vi "Stepper Configure.vi"(7 "Stepper #":u8, 8 "Error In":errorcluster, 9 "Control Method":T4=enum."2 Wire", 10 "Stepper Pins":u8[](array[numeric]), 11 "ChipKit Resource":T1={"COM Port"="", "Board Type"=enum."ChipKit uC32", "Connection Type"=enum."USB / Serial", "Baud Rate (115200)"=15, "Bytes Per Packet (15)"=15}) -> (0 "Error Out":errorcluster, 3 "ChipKit Resource":T1={"COM Port"="", "Board Type"=enum."ChipKit uC32", "Connection Type"=enum."USB / Serial", "Baud Rate (115200)"=15, "Bytes Per Packet (15)"=15})   [LabVIEW 2011, in "LabVIEW Interface for ChipKit.lvlib"]
doc: "Specify a stepper #(0-7) and the digital pins for H-bridge based or step & direction stepper drivers. Specify a stepper #(0-1) without pins for use with the Adafruit Motor Shield."
uses:
  LabVIEW Interface for ChipKit.lvlib
  Private/Type Defs/Stepper Control Method.ctl
  Private/Type Defs/Chipkit Resource.ctl
  Private/Type Defs/Board Type.ctl
  Private/Type Defs/Connection Type.ctl
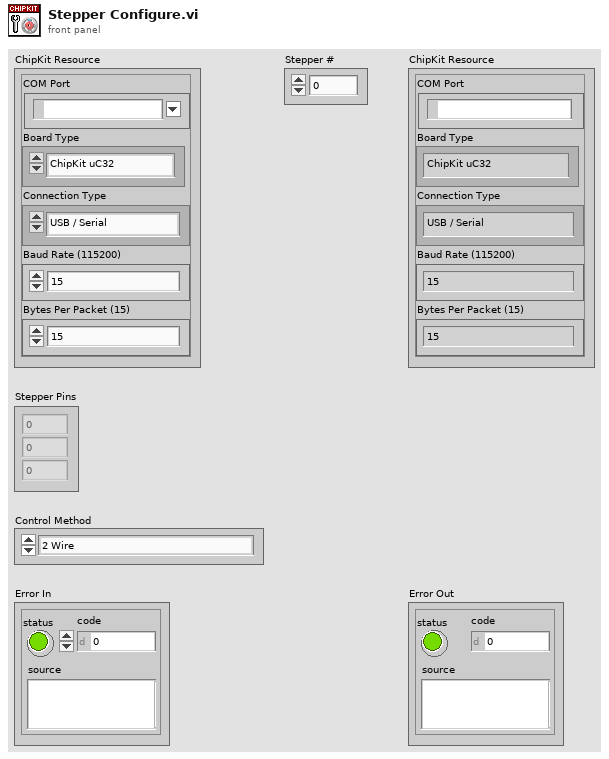
[diagram p1: front panel]
types:
  T1 = typedef "LabVIEW Interface for ChipKit.lvlib/Chipkit Resource.ctl" = cluster{"COM Port":refnum<visa-resource-name>, "Board Type":T2, "Connection Type":T3, "Baud Rate (115200)":u32, "Bytes Per Packet (15)":u32}
  T2 = typedef "LabVIEW Interface for ChipKit.lvlib/Board Type.ctl" = enum16{"ChipKit uC32", "ChipKit Uno32", "ChipKit Max32"}
  T3 = typedef "LabVIEW Interface for ChipKit.lvlib/Connection Type.ctl" = enum8{"USB / Serial", "XBEE", "BlueSmirf (Bluetooth)"}
  T4 = typedef "LabVIEW Interface for ChipKit.lvlib/Stepper Control Method.ctl" = enum16{"2 Wire (Pulse & Direction)", "2 Wire", "4 Wire", "EasyDriver", "AF Motor Shield (Stepper 1 & 2 Only)"}
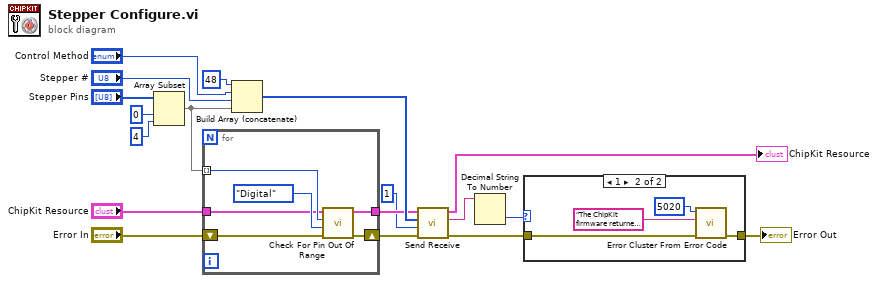
[diagram p0: block diagram]
diagram:
  n1 = Array Subset(array="Stepper Pins", index=0, length=4) -> (w11:u8[])
  n2 = for {
    tunnel: w11 -> [w24] mode=indexing
    tunnel: "ChipKit Resource" -> [w22]
    tunnel: [w21] -> w5
    shift-right: [w19] -> w3
    shift-left: "Error In" -> [w20]
    n3 = call "Check For Pin Out Of Range.vi"("Error In"=w20, "Pin Type"=enum16{"Analog", "Digital"}."Digital", "User Pin Number"=w24, "Arduino Resource"=w22) -> ("Error Out"=w19:errorcluster, "Arduino Resource"=w21:T1)  [unwired: 6 in]
  }
  n4 = Build Array (concatenate)(u8 48, "Control Method", "Stepper #", w11) -> (w8:u16[])
  n5 = call "Send Receive.vi"("Error In"=w3, "Bytes To Read (0)"=u8 1, "Data"=w8, "ChipKit Resource"=w5) -> ("Error Out"=w6:errorcluster, "Read Buffer"=w4:string, "ChipKit Resource"=→"ChipKit Resource":T1)  [unwired: 5 in]
  n6 = Decimal String To Number(string=w4) -> (number=w9:i32)  [unwired: 2 in, 1 out]
  n7 = case shown="1" w9 {
    tunnel: w6 -> [w25 w27]
    tunnel: [w25 w26] -> w10
    frame 0, Default {
    }
    frame 1 {
      n8 = call <vilib>:"Error Cluster From Error Code.vi"("error in (no error)"=w27, "error message (\"\")"="The ChipKit firmware returned an error when attempting to apply the stepper motor configuration." ("source"), "error code (0)"=5020) -> ("error out"=w26:errorcluster)  [unwired: 6 in]
    }
  }
  "Error Out" <- w10
